vi "Test Program  Updated.vi"(11 "VICI Settings":T1) -> ()   [LabVIEW 2018, in "VICI M6 M50 Party Mode.lvlib"]
uses:
  VICI M6 M50 Party Mode.lvlib
  Settings Cluster.ctl
  <vilib>/Instr/_visa.llb/VISA Find Search Mode.ctl
  VICI Global.ctl
  <vilib>/Platform/TimedLoop/XDataNode/timing_clust.ctl
  <vilib>/Platform/TimedLoop/XDataNode/nitl_modes.ctl
  <vilib>/Platform/TimedLoop/XDataNode/wakeup.ctl
  <vilib>/Platform/TimedLoop/XDataNode/XDataNode.xnode
  VICI Global Library.lvlib
  support/Support Library.lvlib
  <vilib>/Platform/TimedLoop/XDataNode/XDNodeRunTimeDep.lvlib
panel:
  out "Initialized":bool
  out "Pump On?":enum16{"Off", "On", "Not Initialized"}(ring)
  in  "stop":bool
  in  "speed":dbl
  # "Pump Head Vol for M6 = 100\nPump Head Vol for M50 = 625"
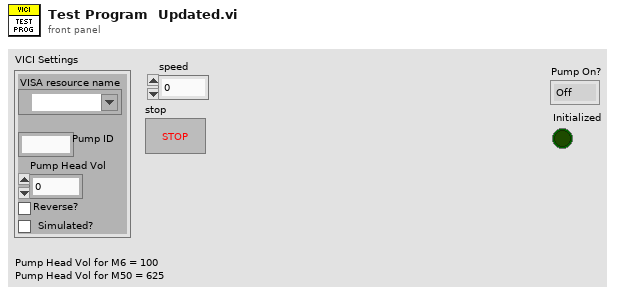
[diagram p1: front panel]
types:
  T1 = typedef "VICI M6 M50 Party Mode.lvlib/Settings Cluster.ctl" = cluster{"VISA resource name":refnum<visa-resource-name>, "Pump ID":string, "Pump Head Vol":dbl, "Reverse?":bool, "Simulated?":bool}
  T2 = typedef "VISA Find Search Mode.ctl" = u32
  T3 = typedef "VICI M6 M50 Party Mode.lvlib/VICI Global Library.lvlib/VICI Global.ctl" = cluster{"Busy":bool, "VISA #":string, "Current Pump":string, "Current Function":string, "Pump Array":string[], "Last Success":timestamp, "ID Queue":string[]}
  T4 = typedef "XDNodeRunTimeDep.lvlib/timing_clust.ctl" = cluster{"Expected End [f-1]":u64, "Actual End [f-1]":u64, "Finished Late? [f-1]":bool, "Expected End [i-1]":u64, "Actual End [i-1]":u64, "Finished Late? [i-1]":bool, "Expected Start [i]":u64, "Actual Start [i]":u64, "Expected Start [f]":u64, "Actual Start [f]":u64, "Source Name":string, "Structure Name":string, "Period":i64, "Deadline":i64, "Offset":i64, "Start":i64, "Priority":i32, "Timeout":i32, "Mode":T5, "Wakeup Reason":T6, "Error":errorcluster, "Source Type":string, "Secondary Source Type":string, "Global End Time":u64, "Global Start Time":u64, "Frame Duration":u64, "Iteration Duration":u64, "Assigned CPU":i32, "I/O Scan Engine Mode":u32}
  T5 = typedef "XDNodeRunTimeDep.lvlib/nitl_modes.ctl" = enum32{"No Change", "Process missed periods, maintain original phase", "Discard missed periods, maintain original phase", "Process missed periods, ignore original phase", "Discard missed periods, ignore original phase"}
  T6 = typedef "XDNodeRunTimeDep.lvlib/wakeup.ctl" = enum32{"Normal", "Aborted", "Asynchronous wakeup", "Timing source error", "Timed loop error", "Timeout"}
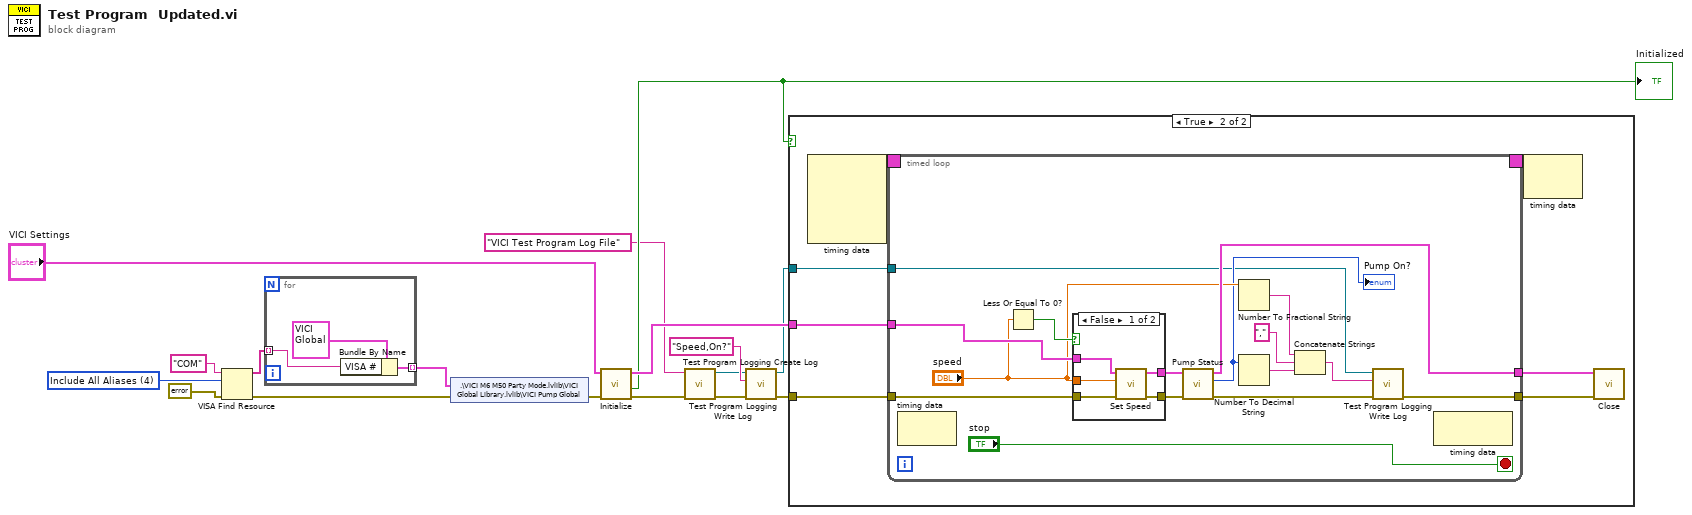
[diagram p0: block diagram]
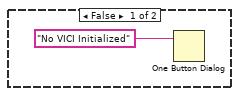
[diagram p2: hidden frame]
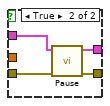
[diagram p3: hidden frame]
diagram:
  w10 = T2 4 items=["Canonical Names Only"=0, "Aliases Only"=2, "Include Matching Aliases"=3, "Include All Aliases"=4] ("Search Mode")
  n1 = VISA Find Resource(8:errorcluster {"status"=FALSE, "code"=0, "source"=""} ("error in (no error)"), 10:w10, 11:"COM" ("expression (\"?*\")")) -> (0:w12:errorcluster, 3:w14:string[])  [unwired: 1 out]
  n2 = for {
    tunnel: w14 -> [w19] mode=indexing
    tunnel: [w18] -> w13 mode=indexing
    n3 = Bundle By Name(cluster=T3 {"Busy"=FALSE, "VISA #"="", "Current Pump"="", "Current Function"="", "Pump Array"=[], "Last Success"=timestamp(0 s since 1904-01-01), "ID Queue"=[]} ("VICI Global"), "VISA #"=w19) -> (w18:T3)
  }
  n4 = shared-variable ".\\VICI M6 M50 Party Mode.lvlib\\VICI Global Library.lvlib\\VICI Pump Global"(w13, error in=w12) -> (error out=w9:errorcluster)
  n5 = call "Initialize.vi"("error in (no error)"=w9, "VICI Settings"="VICI Settings") -> ("error out"=w8:errorcluster, "Initialized"=w16:bool, "VICI Settings"=w17:T1)  [unwired: 6 in, 1 out]
  "Initialized" <- w16
  n6 = call "Test Program Logging Create Log.vi"("error in"=w8, "File Name"="VICI Test Program Log File" ("string")) -> ("error out"=w7:errorcluster, "refnum out"=w1:refnum<file>)  [unwired: 8 in]
  n7 = call "Test Program Logging Write Log.vi"("error in"=w7, "text"="Speed,On?", "Test Program Log File"=w1) -> ("error out"=w6:errorcluster, "refnum out"=w3:refnum<file>)  [unwired: 7 in]
  n8 = case shown="True" w16 {
    tunnel: w17 -> [_ w28]
    tunnel: w6 -> [_ w26]
    tunnel: w3 -> [_ w22]
    frame False {
      n9 = One Button Dialog(message="No VICI Initialized") -> ()  [unwired: 1 in, 1 out]
    }
    frame True {
      n10 = node-c288() -> (w24:T4)  [unwired: 4 in]
      n11 = timed-loop {
        tunnel: w28 -> [w40]
        tunnel: [w43] -> w27
        tunnel: w26 -> [w42]
        tunnel: [w37] -> w25
        timing: w24 -> [_]
        timing-out: [_] -> w23
        tunnel: w22 -> [w29]
        stop <- "stop" stop-if-true
        n12 = node-c288() -> ()  [unwired: 1 in, 1 out]
        n13 = Less Or Equal To 0?(x="speed") -> (x <= 0?=w39:bool)
        n14 = case shown="False" w39 {
          tunnel: w40 -> [w51 w55]
          tunnel: [w50 w54] -> w44
          tunnel: w42 -> [w48 w53]
          tunnel: [w49 w52] -> w41
          tunnel: "speed" -> [w47 _]
          frame False {
            n15 = call "Set Speed.vi"("error in (no error)"=w48, "Flow Rate (mL/min)"=w47, "VICI Settings In"=w51) -> ("error out"=w49:errorcluster, "VICI Settings Out"=w50:T1)  [unwired: 6 in, 1 out]
          }
          frame True {
            n16 = call "Pause.vi"("error in (no error)"=w53, "VICI Settings In"=w55) -> ("error out"=w52:errorcluster, "VICI Settings Out"=w54:T1)  [unwired: 7 in, 1 out]
          }
        }
        n17 = call "Pump Status.vi"("error in (no error)"=w41, "VICI Settings In"=w44) -> ("error out"=w38:errorcluster, "Pump On?"=w32:enum16{"Off", "On", "Not Initialized"}, "VICI Settings Out"=w43:T1)  [unwired: 6 in, 1 out]
        "Pump On?" <- w32
        n18 = Number To Fractional String(number="speed") -> (F-format string=w35:string)  [unwired: 3 in]
        n19 = Number To Decimal String(number=w32) -> (decimal integer string=w31:string)  [unwired: 1 in]
        n20 = Concatenate Strings(w35, "," ("string"), w31) -> (w30:string)
        n21 = call "Test Program Logging Write Log.vi"("error in"=w38, "text"=w30, "Test Program Log File"=w29) -> ("error out"=w37:errorcluster)  [unwired: 7 in, 1 out]
        n22 = node-c288() -> ()  [unwired: 1 in, 1 out]
      }
      n23 = node-c288(w23) -> ()  [unwired: 1 out]
      n24 = call "Close.vi"("error in (no error)"=w25, "VICI Settings"=w27) -> ()  [unwired: 7 in, 3 out]
    }
  }
